vi "TETRIX DC Motor Stop_HT_myRIO.vi"(0 "Stop (Brake or Coast)":string(combo)="Brake", 2 "Motor Channel: (1 or 2)":u8=1, 3 "Controller Daisy Chain Position: 1 - 4":u8=1, 4 "error in (no error)":errorcluster) -> (1 "error out":errorcluster)   [LabVIEW 2013]
uses:
  <vilib>/myRIO/Instrument Drivers/Onboard IO/I2C/vis/Smart Open.vi
  <vilib>/myRIO/Instrument Drivers/Onboard IO/I2C/vis/Configure.vi
  <vilib>/myRIO/Instrument Drivers/Onboard IO/I2C/vis/Write.vi
  <vilib>/myRIO/Instrument Drivers/Onboard IO/I2C/vis/Open.vi
  <vilib>/myRIO/Common/Instrument Driver Framework/myRIO v1.0/I2C/vis/myRIO v1.1 Open I2C.vi
  <vilib>/myRIO/Common/Instrument Driver Framework/Utilities/vis/Validate Channels.vi
  <vilib>/myRIO/Common/Instrument Driver Framework/myRIO v1.0/I2C/vis/myRIO v1.0 Reserve I2C.vi
  <vilib>/myRIO/Common/Instrument Driver Framework/myRIO v1.0/I2C/vis/myRIO v1.0 Build MUX Configuration I2C.vi
  <vilib>/myRIO/Common/Instrument Driver Framework/myRIO v1.0/Resource Manager/vis/myRIO v1.0 Reserve Channel List.vi
  <vilib>/myRIO/Common/Instrument Driver Framework/myRIO v1.0/Resource Manager/vis/myRIO v1.0 Create Configuration List.vi
  <vilib>/myRIO/Common/Instrument Driver Framework/myRIO v1.0/Resource Manager/vis/myRIO v1.0 Reserve Channel.vi
  <vilib>/myRIO/Common/Instrument Driver Framework/myRIO v1.0/Resource Manager/vis/myRIO v1.0 Unreserve Channel.vi
  <vilib>/myRIO/Common/Instrument Driver Framework/myRIO v1.0/Resource Manager/vis/myRIO v1.0 Build Mutex Name.vi
  <vilib>/myRIO/Common/Instrument Driver Framework/myRIO v1.0/myRIO v1.1 Open.vi
  <vilib>/Utility/VariantDataType/GetNumericInfo.vi
  <vilib>/Utility/error.llb/Error Cluster From Error Code.vi
  <vilib>/myRIO/Common/Instrument Driver Framework/Utilities/vis/IO Manager.vi
  <vilib>/myRIO/Common/Instrument Driver Framework/Utilities/vis/Configuration Manager.vi
  <vilib>/myRIO/Common/Instrument Driver Framework/myRIO v1.0/Resource Manager/vis/myRIO v1.0 Configure IO.vi
  <vilib>/myRIO/Common/Instrument Driver Framework/myRIO v1.0/myRIO v1.0 Close.vi
  <vilib>/myRIO/Common/Instrument Driver Framework/myRIO v1.0/I2C/vis/myRIO v1.0 Configure I2C.vi
  <vilib>/myRIO/Common/Instrument Driver Framework/myRIO v1.0/I2C/vis/myRIO v1.0 Write I2C.vi
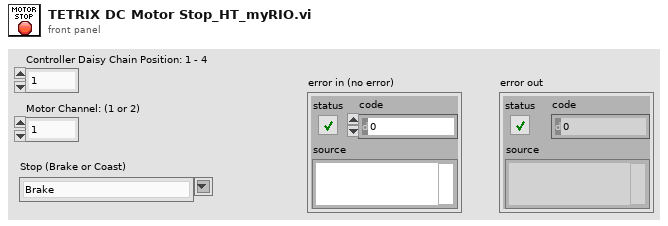
[diagram p1: front panel]
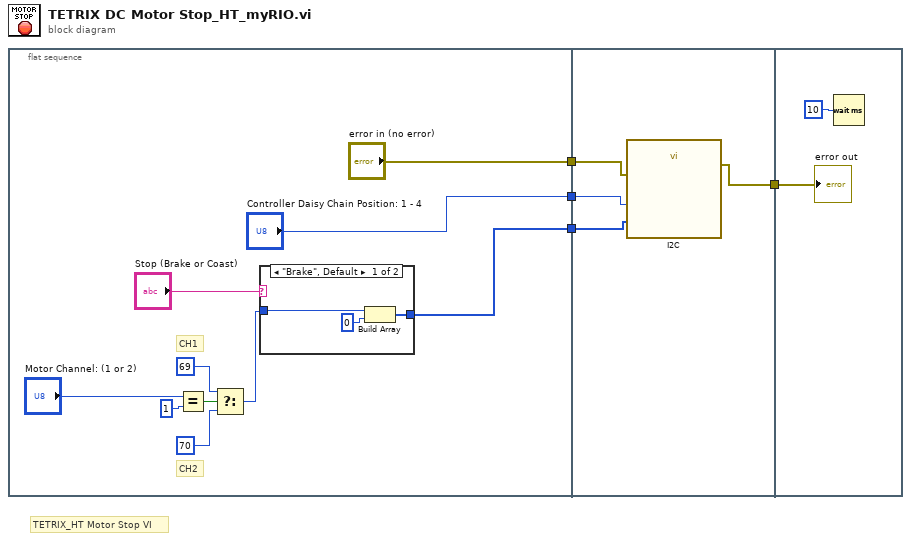
[diagram p0: block diagram]
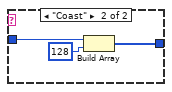
[diagram p2: hidden frame]
diagram:
  # "TETRIX_HT Motor Stop VI"
  n1 = flat-sequence {
    tunnel: ["Controller Daisy Chain Position: 1 - 4"] -> w4
    tunnel: [w6] -> w3
    tunnel: ["error in (no error)"] -> w2
    tunnel: w4 -> [w24]
    tunnel: w3 -> [w23]
    tunnel: w2 -> [w22]
    tunnel: [w21] -> w1
    tunnel: w1 -> [w25]
    frame #0 {
      # "CH2"
      # "CH1"
      n2 = Equal?(x="Motor Channel: (1 or 2)", y=u8 1) -> (x = y?=w11:bool)
      n3 = Select(t=u8 69, s=w11, f=u8 70) -> (s? t:f=w14:u8)
      n4 = case shown="\"Brake\", Default" "Stop (Brake or Coast)" {
        tunnel: w14 -> [w17 w20]
        tunnel: [w15 w18] -> w6
        frame "Brake", Default {
          n5 = Build Array(w17, u8 0 ("element")) -> (w15:u8[])
        }
        frame "Coast" {
          n6 = Build Array(w20, u8 128 ("element")) -> (w18:u8[])
        }
      }
    }
    frame #1 {
      n7 = call "I2C"("Slave Address (7-bit)"=w24, "Bytes to Write"=w23, "error in (no error)"=w22) -> ("error out"=w21:errorcluster)  [unwired: 24 in]
    }
    frame #2 {
      n8 = Wait (ms)(milliseconds to wait=u32 10) -> ()  [unwired: 1 out]
      "error out" <- w25
    }
  }
